vi "LibManager.vi"(7 "action":enum16{"LibInit", "LibExit"}(ring), 8 "error in (no error)":errorcluster) -> (0 "error out":errorcluster, 1 "NuOfServers":u32, 3 "instances count":i32)   [LabVIEW 2020, in "AIM664LV.lvlib"]
doc: "Instantiates a reference to the driver and manages to obtain only one reference to the library. Use <LibInit> wherever you start to reference the library and use <LibExit> after you are done with the specific reference."
uses:
  AIM664LV.lvlib
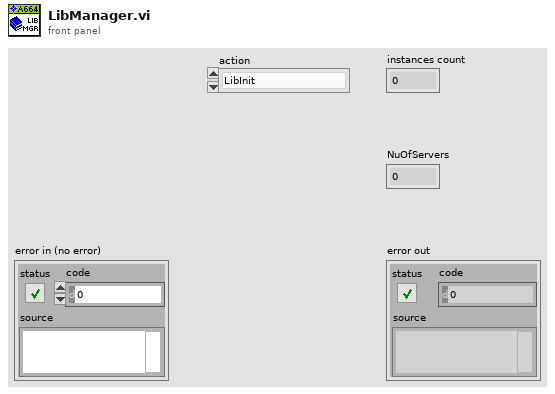
[diagram p1: front panel]
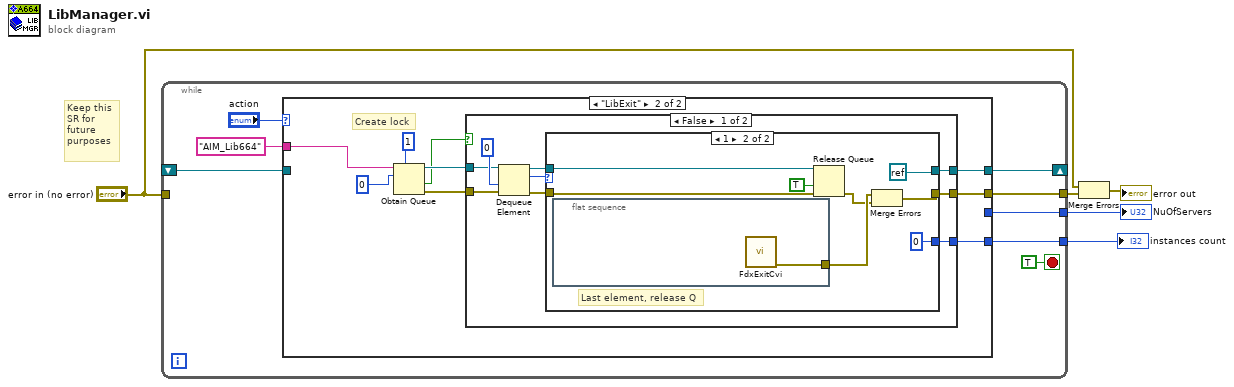
[diagram p0: block diagram]
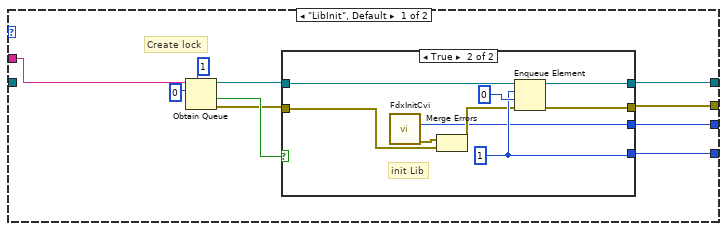
[diagram p2: hidden frame]
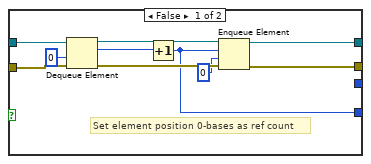
[diagram p3: hidden frame]
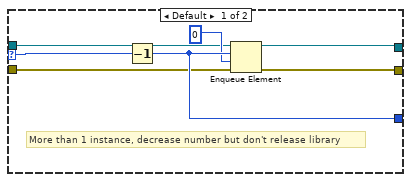
[diagram p4: hidden frame]
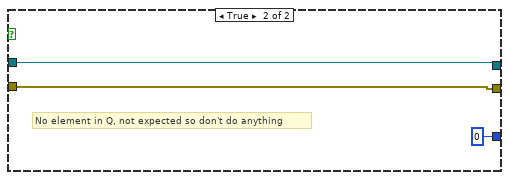
[diagram p5: hidden frame]
diagram:
  # "Keep this \nSR for\nfuture \npurposes"
  n1 = while {
    shift-right: [w10] -> _
    shift-left: _ -> [w9]
    tunnel: [w11] -> w3
    tunnel: [w8] -> w5
    tunnel: [w7] -> w4
    tunnel: "error in (no error)" -> [_]
    stop <- TRUE stop-if-true
    n2 = case shown="\"LibExit\"" "action" {
      tunnel: [w23 w51] -> w11
      tunnel: [w22 w50] -> w10
      tunnel: w9 -> [_ _]
      tunnel: [w21 w49] -> w8
      tunnel: [w15 _] -> w7
      tunnel: "AIM_Lib664" ("name (unnamed)") -> [w14 w43]
      frame "LibInit", Default {
        # "Create lock"
        n3 = Obtain Queue(max queue size (-1, unlimited)=1, name (unnamed)=w14, element data type=0) -> (queue out=w18:refnum<queue>, created new?=w19:bool, error out=w17:errorcluster)  [unwired: 2 in]
        n4 = case shown="True" w19 {
          tunnel: w17 -> [w32 w36]
          tunnel: [w29 w41] -> w23
          tunnel: [w28 w42] -> w22
          tunnel: [w26 w38] -> w21
          tunnel: w18 -> [w33 w39]
          tunnel: [_ w34] -> w15
          frame False {
            # "Set element position 0-bases as ref count"
            n5 = Dequeue Element(queue=w33, timeout in ms (-1)=0, error in (no error)=w32) -> (queue out=w31:refnum<queue>, element=w25:i32, error out=w30:errorcluster)  [unwired: 1 out]
            n6 = Increment(x=w25) -> (x+1=w26:i32)
            n7 = Enqueue Element(queue=w31, element=w26, timeout in ms (-1)=0, error in (no error)=w30) -> (queue out=w28:refnum<queue>, error out=w29:errorcluster)  [unwired: 1 out]
          }
          frame True {
            w38 = 1 ("modules found")
            # "init Lib"
            n8 = call "FdxInitCvi.vi"() -> ("error out"=w35:errorcluster, "Number of Servers"=w34:u32)  [unwired: 10 in]
            n9 = Merge Errors(w35, w36) -> (w37:errorcluster)
            n10 = Enqueue Element(queue=w39, element=w38, timeout in ms (-1)=0, error in (no error)=w37) -> (queue out=w42:refnum<queue>, error out=w41:errorcluster)  [unwired: 1 out]
          }
        }
      }
      frame "LibExit" {
        # "Create lock"
        n11 = Obtain Queue(max queue size (-1, unlimited)=1, name (unnamed)=w43, element data type=0) -> (queue out=w46:refnum<queue>, created new?=w45:bool, error out=w44:errorcluster)  [unwired: 2 in]
        n12 = case shown="False" w45 {
          tunnel: [w60 w77] -> w51
          tunnel: [w59 w78] -> w50
          tunnel: [w58 0] -> w49
          tunnel: w46 -> [w56 w78]
          tunnel: w44 -> [w55 w77]
          frame False {
            n13 = Dequeue Element(queue=w56, timeout in ms (-1)=0, error in (no error)=w55) -> (queue out=w53:refnum<queue>, element=w54:i32, error out=w52:errorcluster)  [unwired: 1 out]
            n14 = case shown="1" w54 {
              selector: w54 -> [w63 _]
              tunnel: [w64 w72] -> w60
              tunnel: [w67 refnum<k0> refnum] -> w59
              tunnel: [w66 0] -> w58
              tunnel: w53 -> [w62 w70]
              tunnel: w52 -> [w61 w69]
              frame Default {
                # "More than 1 instance, decrease number but don't release library"
                n15 = Decrement(x=w63) -> (x-1=w66:i32)
                n16 = Enqueue Element(queue=w62, element=w66, timeout in ms (-1)=0, error in (no error)=w61) -> (queue out=w67:refnum<queue>, error out=w64:errorcluster)  [unwired: 1 out]
              }
              frame 1 {
                # "Last element, release Q"
                n17 = flat-sequence {
                  tunnel: [w76] -> w74
                  frame #0 {
                    n18 = call "FdxExitCvi.vi"() -> ("error out"=w76:errorcluster)  [unwired: 11 in]
                  }
                }
                n19 = Release Queue(queue=w70, force destroy? (F)=TRUE, error in (no error)=w69) -> (error out=w73:errorcluster)  [unwired: 2 out]
                n20 = Merge Errors(w74, w73) -> (w72:errorcluster)
              }
            }
          }
          frame True {
            # "No element in Q, not expected so don't do anything"
          }
        }
      }
    }
  }
  "instances count" <- w5
  "NuOfServers" <- w4
  n21 = Merge Errors("error in (no error)", w3) -> (→"error out":errorcluster)
